vi "Stop PJVS.vi"(8 "error in (pass through)":errorcluster, 11 "PJVS setup":T1={"PJVS type"=enum."AC-supraVOLTcontrol", "Status Refnum"=refnum, "AC-supraVOLTcontrol"={"IP address:port (0.0.0.0:0000)"="0.0.0.0:0000", "Timeouts"={"TCP Read & Write (ms)"=7000, "Sensors readout"=5000, "PJVS setup"=10000, "Nullmeter readout"=5000, "Multiplexer setup"=3000, "57XX setup"=15000, "Generator setup"=5000, "Synthesizer setup"=3000, "Sampler readout"=10000}, "Simulation mode"=FALSE, "Debug mode"=FALSE}, "NPL bias source"={"DataSocketCluster"={"Server Machine"="CZC", "Client Machine"="localhost", "Data"="P2", "TimeStamp"=0.0, "Count"=1, "Target Process"="General Server"}}, "Manual PJVS"={"PJVS frequency (Hz)"=0.0, "Reference voltages (V)"=[], "File with PJVS voltages"=path ""}, "VTT PJVS"={"some VTT only property"=""}} {"NPL bias source"."DataSocketCluster"."TimeStamp" format="%.2f"}) -> (0 "error out":errorcluster, 3 "PJVS setup out":T1={"PJVS type"=enum."AC-supraVOLTcontrol", "Status Refnum"=refnum, "AC-supraVOLTcontrol"={"IP address:port (0.0.0.0:0000)"="0.0.0.0:0000", "Timeouts"={"TCP Read & Write (ms)"=7000, "Sensors readout"=5000, "PJVS setup"=10000, "Nullmeter readout"=5000, "Multiplexer setup"=3000, "57XX setup"=15000, "Generator setup"=5000, "Synthesizer setup"=3000, "Sampler readout"=10000}, "Simulation mode"=FALSE, "Debug mode"=FALSE}, "NPL bias source"={"DataSocketCluster"={"Server Machine"="CZC", "Client Machine"="localhost", "Data"="P2", "TimeStamp"=0.0, "Count"=1, "Target Process"="General Server"}}, "Manual PJVS"={"PJVS frequency (Hz)"=0.0, "Reference voltages (V)"=[], "File with PJVS voltages"=path ""}, "VTT PJVS"={"some VTT only property"=""}} {"NPL bias source"."DataSocketCluster"."TimeStamp" format="%.2f"})   [LabVIEW 2020]
doc: "Stops PJVS. For supracon system, the PJVS is set to 0 V 0 Hz and multiplexer is disconnected. For NPL Bias source, the PJVS is set to 0 V."
uses:
  Type definitions/PJVS.ctl
  Type definitions/PJVS Type.ctl
  external libraries/acsvcontrol-driver/Public/Type Definitions/Timeouts.ctl
  external libraries/JV modified NPL Bias source/DataSocketCluster external.ctl
  external libraries/acsvcontrol-driver/Public/Type Definitions/Multiplexer.ctl
  b78424e6-2e46-4611-a0f5-49ae892956c0.vi
  external libraries/acsvcontrol-driver/ACSVcontrol-driver.lvlib
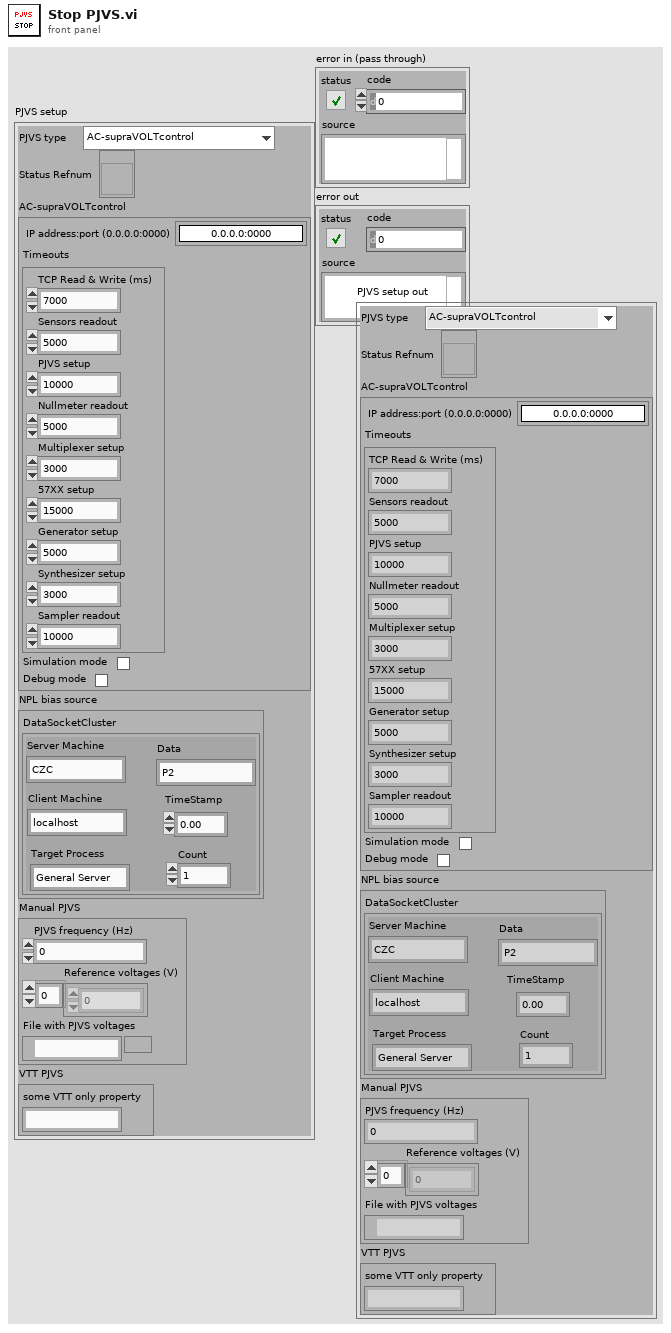
[diagram p1: front panel]
types:
  T1 = typedef "PJVS.ctl" = cluster{"PJVS type":T2, "Status Refnum":refnum<vi>, "AC-supraVOLTcontrol":cluster{"IP address:port (0.0.0.0:0000)":string, "Timeouts":T3, "Simulation mode":bool, "Debug mode":bool}, "NPL bias source":cluster{"DataSocketCluster":T4}, "Manual PJVS":cluster{"PJVS frequency (Hz)":dbl, "Reference voltages (V)":dbl[], "File with PJVS voltages":path}, "VTT PJVS":cluster{"some VTT only property":string}}
  T2 = typedef "PJVS Type.ctl" = enum16{"AC-supraVOLTcontrol", "JV modified NPL bias control", "Manual PJVS", "VTT PJVS"}
  T3 = typedef "ACSVcontrol-driver.lvlib/Timeouts.ctl" = cluster{"TCP Read & Write (ms)":i32, "Sensors readout":i32, "PJVS setup":i32, "Nullmeter readout":i32, "Multiplexer setup":i32, "57XX setup":i32, "Generator setup":i32, "Synthesizer setup":i32, "Sampler readout":i32}
  T4 = typedef "DataSocketCluster external.ctl" = cluster{"Server Machine":string, "Client Machine":string, "Data":string, "TimeStamp":dbl, "Count":i32, "Target Process":string}
  T5 = typedef "ACSVcontrol-driver.lvlib/Multiplexer.ctl" = enum16{"Short DC Nano / Voltmeter", "Short AC Sampler", "Short Switch DC (JVS->Nano)", "Short Switch AC (JVS->Digit)", "JVS-Voltmeter", "Channel A positive", "Channel A negative", "Channel B positive", "Channel B negative", "Channel C positive", "Channel C negative", "Nulldetector-Channel A+", "Nulldetector-Channel A-", "Nulldetector-Channel B+", "Nulldetector-Channel B-", "Nulldetector-Channel C+", "Nulldetector-Channel C-", "ext.Voltmeter-Channel A+", "ext.Voltmeter-Channel A-", "ext.Voltmeter-Channel B+", "ext.Voltmeter-Channel B-", "ext.Voltmeter-Channel C+", "ext.Voltmeter-Channel C-"}
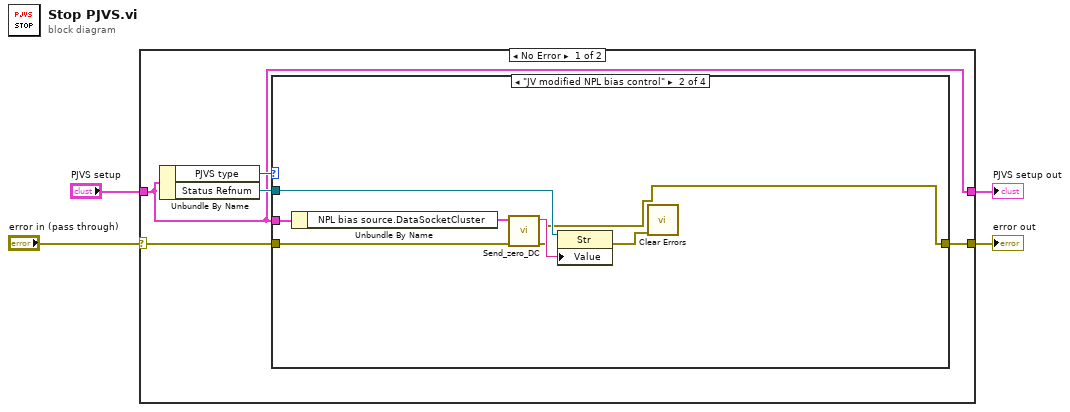
[diagram p0: block diagram]
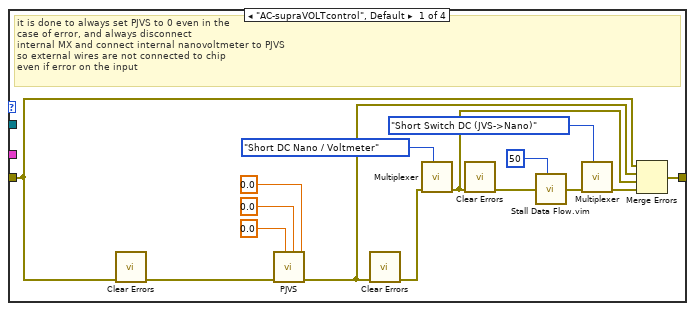
[diagram p2: hidden frame]
diagram:
  n1 = case shown="No Error" "error in (pass through)" {
    selector: "error in (pass through)" -> [w6 w35]
    tunnel: "PJVS setup" -> [w5 w34]
    tunnel: [w7 w35] -> w3
    tunnel: [w5 w34] -> w1
    frame No Error {
      n2 = Unbundle By Name(w5) -> ("PJVS type"=w9:T2, "Status Refnum"=w8:refnum<vi>)
      n3 = case shown="\"JV modified NPL bias control\"" w9 {
        tunnel: w8 -> [_ w27 _ _]
        tunnel: w6 -> [w19 w31 w32 w33]
        tunnel: [w20 w25 w32 w33] -> w7
        tunnel: w5 -> [_ w30 _ _]
        frame "AC-supraVOLTcontrol", Default {
          # "it is done to always set PJVS to 0 even in the \ncase of error, and always disconnect\ninternal MX and connect internal nanovoltmeter to PJVS\nso external wires are not connected to chip\neven if error on the input"
          n4 = call <vilib>:"Clear Errors.vi"("error in (no error)"=w19) -> ("error out"=w18:errorcluster)  [unwired: 5 in, 1 out]
          n5 = call "PJVS.vi"("Trim current (A) (+- 0.002)"=0.0, "Frequency  (0 Hz) (0, 0.5 - 10e3)"=0.0, "Voltage (0 V DC/RMS) (DC: +- 10.1, AC: 0 - 7.2)"=0.0, "error in (no error)"=w18) -> ("error out"=w17:errorcluster)  [unwired: 6 in, 1 out]
          n6 = call <vilib>:"Clear Errors.vi"("error in (no error)"=w17) -> ("error out"=w16:errorcluster)  [unwired: 5 in, 1 out]
          n7 = call "Multiplexer.vi"("Multiplexer (Short DC Nano / Voltmeter)"=Multiplexer."Short DC Nano / Voltmeter", "error in (no error)"=w16) -> ("error out"=w15:errorcluster)  [unwired: 9 in]
          n8 = call <vilib>:"Clear Errors.vi"("error in (no error)"=w15) -> ("error out"=w12:errorcluster)  [unwired: 5 in, 1 out]
          n9 = call "Stall Data Flow.vim"("value in"=w12, "milliseconds to wait"=u32 50) -> ("value out"=w11:errorcluster)  [unwired: 1 out]
          n10 = call "Multiplexer.vi"("Multiplexer (Short DC Nano / Voltmeter)"=Multiplexer."Short Switch DC (JVS->Nano)", "error in (no error)"=w11) -> ("error out"=w13:errorcluster)  [unwired: 9 in]
          n11 = Merge Errors(w19, w17, w15, w13) -> (w20:errorcluster)
        }
        frame "JV modified NPL bias control" {
          n12 = Unbundle By Name(w30) -> ("NPL bias source.DataSocketCluster"=w29:T4)
          n13 = call "Send_zero_DC.vi"("error in (no error)"=w31, "machine"=w29) -> ("error out"=w25:errorcluster, "String"=w28:string)  [unwired: 8 in]
          n14 = property class="Str"(reference=w27, "Value"=w28) -> (error out=w26:errorcluster)  [unwired: 1 in, 1 out]
          n15 = call <vilib>:"Clear Errors.vi"("error in (no error)"=w26) -> ()  [unwired: 5 in, 2 out]
        }
        frame "Manual PJVS" {
          # "#INRIM add something here"
        }
        frame "VTT PJVS" {
          # "#VTT add something here"
        }
      }
    }
    frame Error {
    }
  }
  "error out" <- w3
  "PJVS setup out" <- w1
